vi "IMAQController.ImageProcessing.vi"(0 "i ref in":refnum<vi>, 1 "Image ref in":refnum<vi>, 2 "ActImage":T2, 3 "RawImage":T2, 4 "DIM data":i16[](array[numeric]), 5 "ImageHeight":i32, 6 "ImageWidth":i32, 7 "error in (no error)":errorcluster, 8 "Ana Step 1 Event":refnum<user-event>, 9 "Save?":bool, 10 "Grid Color":u32(colorbox)=16448250, 11 "Overlay Lines In":T4(array[cluster]), 12 "Save path in":path, 13 "Overlay already configured?":bool, 14 "Save Overlay?":bool, 15 "ShowGrid?":bool, 16 "Scan Variables":T1, 17 "SaveImage":T2, 18 "Scan Running?":bool, 19 "Averaging":u8=1) -> (20 "i ref out":refnum<vi>, 22 "Overlay Lines Out":T4(array[cluster]), 23 "ActImage Out":T2, 24 "Error?":bool, 25 "AverageString":string, 27 "error out":errorcluster)   [LabVIEW 2014, in "IMAQController.lvlib"]
uses:
  IMAQController.lvlib
  <vilib>/vision/Image Controls.llb/IMAQ Image.ctl
panel:
  out "activeCamera.Aqcuisation Mode":T3(ring)
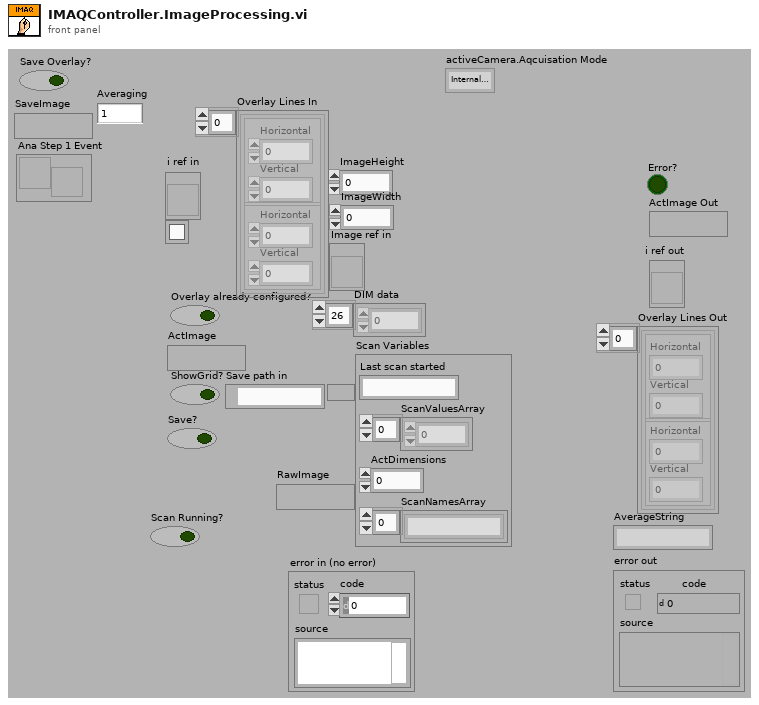
[diagram p1: front panel]
types:
  T1 = cluster{"Last scan started":string, "ScanValuesArray":dbl[], "ActDimensions":i16, "ScanNamesArray":string[]}
  T2 = typedef "IMAQ Image.ctl" = refnum<image>
  T3 = enum32{"Internal Trigger", "Scan", "free Running", "External Trigger"}
  T4 = cluster{cluster{"Horizontal":i32, "Vertical":i32}, cluster{"Horizontal":i32, "Vertical":i32}}[]
  T5 = enum32{"Gray", "Binary", "Gradient", "Rainbow", "Temperature"}
  T6 = typedef "IMAQController.lvlib/IMAQController.i attribute.ctl" = cluster{"ImageTakenID":i32, "actSequencer":string, "actScanner":string, "CameraTriggerID":i32, "activatedCameras":cluster{"Name":string, "Camera Type":string, "Acquisition Mode":u32, "JPEG Mode?":bool, "Acquisition Delay":dbl, "Save Images?":bool, "Center Coordinates":T7, "PixelPermm":cluster{"Horizontal":dbl, "Vertical":dbl}, "Rotation":dbl, "Mirror Mode":u32, "PixelCoordinates":cluster{"1":cluster{"Horizontal":i32, "Vertical":i32}, "2":cluster{"Horizontal":i32, "Vertical":i32}, "3":cluster{"Horizontal":i32, "Vertical":i32}, "4":cluster{"Horizontal":i32, "Vertical":i32}}, "RWCoordinates":cluster{"1":cluster{"Horizontal":dbl, "Vertical":dbl}, "2":cluster{"Horizontal":dbl, "Vertical":dbl}, "3":cluster{"Horizontal":dbl, "Vertical":dbl}, "4":cluster{"Horizontal":dbl, "Vertical":dbl}}, "HorizScaling":dbl, "VertScaling":dbl}[], "Ini C-Array":string[], "actCamera":string, "activeCamera":cluster{"Name":string, "Camera Type":string, "Aqcuisation Mode":enum32{"Internal Trigger", "Scan", "free Running", "External Trigger"}, "JPEG Mode?":bool, "Acquisition Delay":dbl, "Save Images?":bool, "Center Coordinates":T7, "PixelPermm":cluster{"Horizontal":dbl, "Vertical":dbl}, "Rotation":dbl, "Mirror Mode":u32, "PixelCoordinates":cluster{"1":cluster{"Horizontal":i32, "Vertical":i32}, "2":cluster{"Horizontal":i32, "Vertical":i32}, "3":cluster{"Horizontal":i32, "Vertical":i32}, "4":cluster{"Horizontal":i32, "Vertical":i32}}, "RWCoordinates":cluster{"1":cluster{"Horizontal":dbl, "Vertical":dbl}, "2":cluster{"Horizontal":dbl, "Vertical":dbl}, "3":cluster{"Horizontal":dbl, "Vertical":dbl}, "4":cluster{"Horizontal":dbl, "Vertical":dbl}}, "HorizScaling":dbl, "VertScaling":dbl}, "BilderMittelungen":u8, "OldPicture":dbl[][]}
  T7 = typedef "LVPoint32TypeDef.ctl" = cluster{"Horizontal":i32, "Vertical":i32}
  T8 = cluster{"Name":string, "Camera Type":string, "Acquisition Mode":u32, "JPEG Mode?":bool, "Acquisition Delay":dbl, "Save Images?":bool, "Center Coordinates":T7, "PixelPermm":cluster{"Horizontal":dbl, "Vertical":dbl}, "Rotation":dbl, "Mirror Mode":u32, "PixelCoordinates":cluster{"1":cluster{"Horizontal":i32, "Vertical":i32}, "2":cluster{"Horizontal":i32, "Vertical":i32}, "3":cluster{"Horizontal":i32, "Vertical":i32}, "4":cluster{"Horizontal":i32, "Vertical":i32}}, "RWCoordinates":cluster{"1":cluster{"Horizontal":dbl, "Vertical":dbl}, "2":cluster{"Horizontal":dbl, "Vertical":dbl}, "3":cluster{"Horizontal":dbl, "Vertical":dbl}, "4":cluster{"Horizontal":dbl, "Vertical":dbl}}, "HorizScaling":dbl, "VertScaling":dbl}[]
  T9 = cluster{"Name":string, "Camera Type":string, "Acquisition Mode":u32, "JPEG Mode?":bool, "Acquisition Delay":dbl, "Save Images?":bool, "Center Coordinates":T7, "PixelPermm":cluster{"Horizontal":dbl, "Vertical":dbl}, "Rotation":dbl, "Mirror Mode":u32, "PixelCoordinates":cluster{"1":cluster{"Horizontal":i32, "Vertical":i32}, "2":cluster{"Horizontal":i32, "Vertical":i32}, "3":cluster{"Horizontal":i32, "Vertical":i32}, "4":cluster{"Horizontal":i32, "Vertical":i32}}, "RWCoordinates":cluster{"1":cluster{"Horizontal":dbl, "Vertical":dbl}, "2":cluster{"Horizontal":dbl, "Vertical":dbl}, "3":cluster{"Horizontal":dbl, "Vertical":dbl}, "4":cluster{"Horizontal":dbl, "Vertical":dbl}}, "HorizScaling":dbl, "VertScaling":dbl}
  T10 = cluster{"Data":u8[][], "Height":i32, "Width":i32, "Save path out Scan":path, "Save path out Horizontal":path, "Save path out Vertical":path, "Scan?":bool, "Scan running?":bool, "ScanValuesArray":dbl[], "ActDimensions":i16, "ScanNamesArray":string[], "Av repeat?":bool}
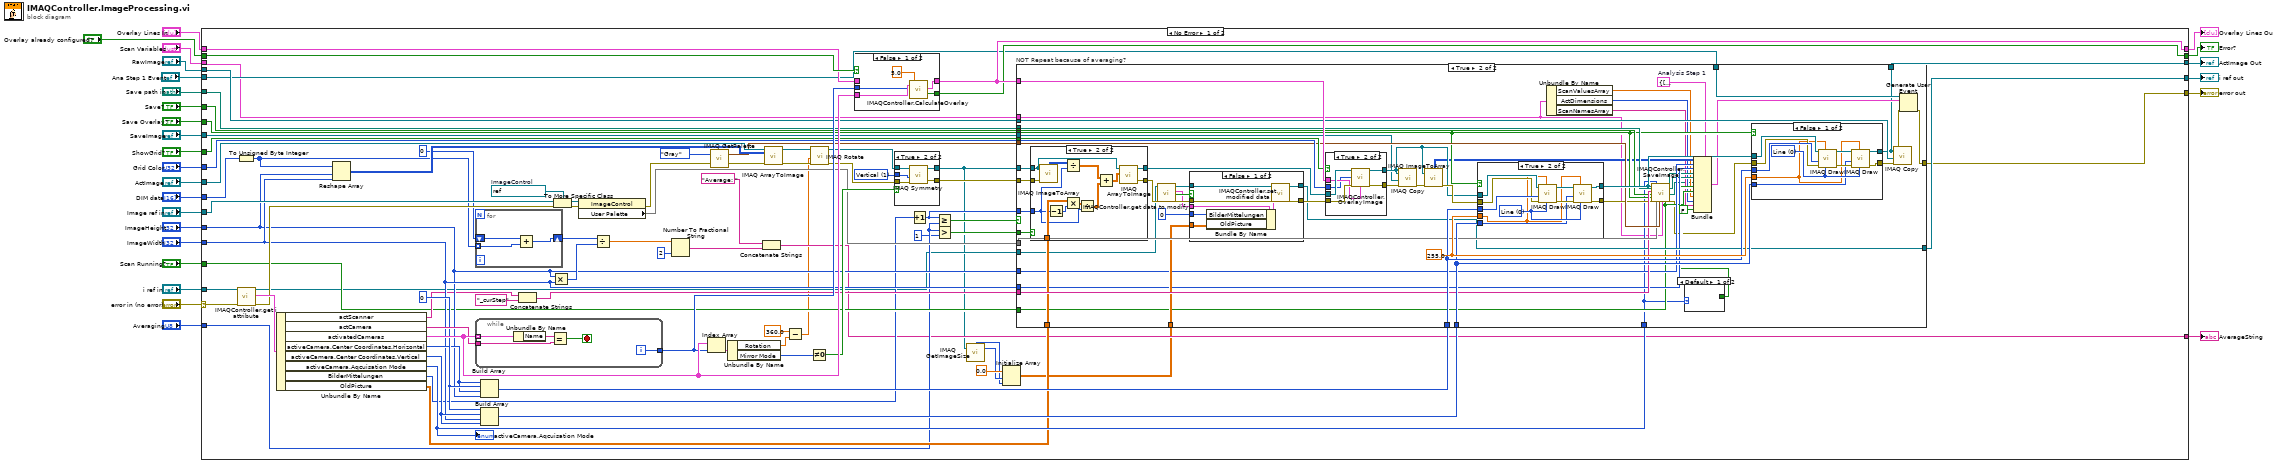
[diagram p0: block diagram]
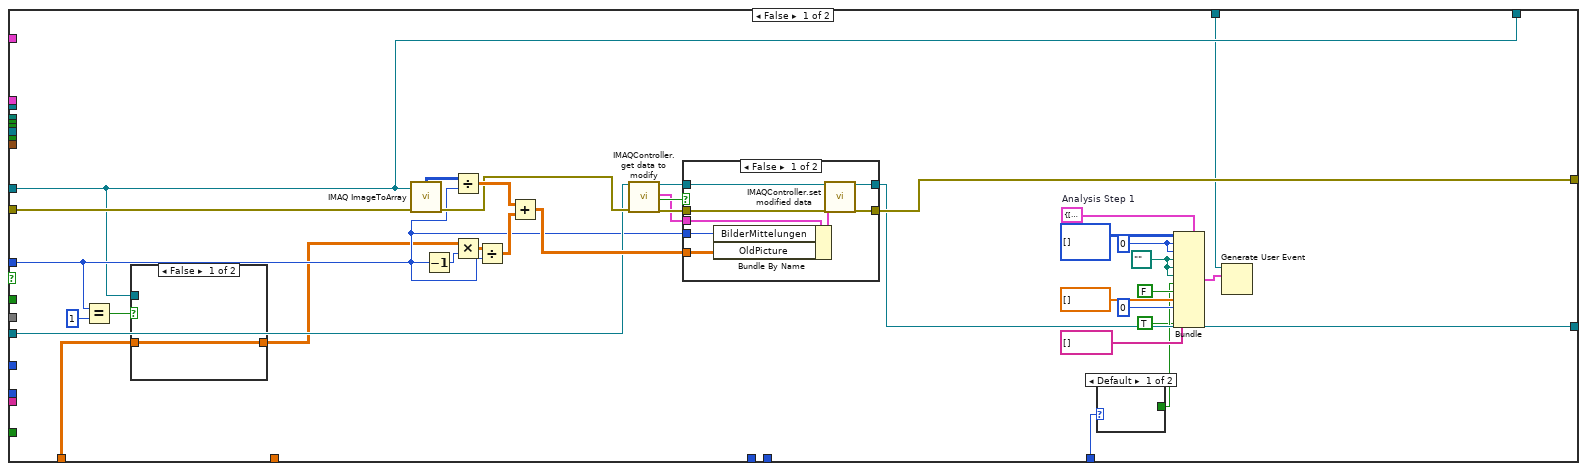
[diagram p2: hidden frame]
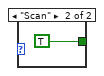
[diagram p3: hidden frame]
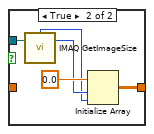
[diagram p4: hidden frame]
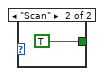
[diagram p6: hidden frame]
diagram:
  n1 = case shown="No Error" "error in (no error)" {
    selector: "error in (no error)" -> [w69 w297]
    tunnel: "i ref in" -> [w106 w296]
    tunnel: "Overlay already configured?" -> [w105 _]
    tunnel: "Overlay Lines In" -> [w104 _]
    tunnel: "Image ref in" -> [w103 _]
    tunnel: "DIM data" -> [w93 _]
    tunnel: "Grid Color" -> [w83 _]
    tunnel: [w82 _] -> w20
    tunnel: "ShowGrid?" -> [w81 _]
    tunnel: "Save path in" -> [w56 _]
    tunnel: "ImageHeight" -> [w61 _]
    tunnel: "ImageWidth" -> [w62 _]
    tunnel: [w39 _] -> w15
    tunnel: "RawImage" -> [w70 _]
    tunnel: [w32 w297] -> w13
    tunnel: "ActImage" -> [w68 w295]
    tunnel: [w33 w296] -> w10
    tunnel: [w59 w295] -> w9
    tunnel: "Save?" -> [w52 _]
    tunnel: [w66 _] -> w7
    tunnel: "Save Overlay?" -> [w51 _]
    tunnel: "SaveImage" -> [w49 _]
    tunnel: "Scan Variables" -> [w30 _]
    tunnel: "Scan Running?" -> [w48 _]
    tunnel: "Averaging" -> [w44 _]
    tunnel: "Ana Step 1 Event" -> [w31 _]
    frame No Error {
      w65 = 0 ("element")
      w87 = u32 1 items=["Horizontal", "Vertical", "Central", "1st Diagonal", "2nd Diagonal"] ("Type of Symmetry")
      w102 = refnum<vi> refnum  # ImageControl
      n2 = To Unsigned Byte Integer(number=w93) -> (unsigned 8bit integer=w71:u8[])
      n3 = call "IMAQController.get i attribute.vi"("i ref in"=w106, "error in (no error)"=w69) -> ("i ref out"=w40:refnum<vi>, "i attribute"=w107:T6, "error out"=w100:errorcluster)  [unwired: 15 in]
      n4 = Unbundle By Name(w107) -> ("actScanner"=w60:string, "actCamera"=w80:string, "activatedCameras"=w92:T8, "activeCamera.Center Coordinates.Horizontal"=w64:i32, "activeCamera.Center Coordinates.Vertical"=w63:i32, "activeCamera.Aqcuisation Mode"=w50:T3, "BilderMittelungen"=w45:u8, "OldPicture"=w46:dbl[][])
      "activeCamera.Aqcuisation Mode" <- w50
      n5 = Reshape Array(w71, w61, w62) -> (w94:u8[][])
      n6 = for {
        tunnel: w71 -> [w281] mode=indexing
        shift-right: [w280] -> w77
        shift-left: 0 -> [w282]
        n7 = Add(x=w282, y=w281) -> (x+y=w280:i32)
      }
      n8 = while {
        tunnel: w92 -> [w291] mode=indexing
        tunnel: w80 -> [w294]
        tunnel: [w292] -> w91
        i -> [w292]
        stop <- w293 stop-if-true
        n9 = Unbundle By Name(w291) -> ("Name"=w290:string)
        n10 = Equal?(x=w290, y=w294) -> (x = y?=w293:bool)
      }
      n11 = Build Array(w64, w65, w64, w61) -> (w58:i32[])
      n12 = Build Array(w65, w63, w62, w63) -> (w57:i32[])
      n13 = Concatenate Strings(w60, "_curStep" ("string")) -> (w53:string)
      n14 = Multiply(x=w61, y=w62) -> (x*y=w75:i32)
      n15 = To More Specific Class(target class=w102, reference=w103, error in=w100) -> (specific class reference=w101:refnum<vi>, error out=w99:errorcluster)
      n16 = property on="Property Node" class="ImageControl"(reference=w101, error in=w99) -> (error out=w97:errorcluster, "User Palette"=w54)  [unwired: 1 out]
      n17 = Divide(x=w77, y=w75) -> (x/y=w76:dbl)
      n18 = Number To Fractional String(number=w76, precision (6)=i16 2 ("width (-)")) -> (F-format string=w73:string)  [unwired: 2 in]
      n19 = Index Array(array=w92, index=w91) -> (element=w90:T9)
      n20 = call "IMAQ GetPalette"("Palette Number (gray)"=T5."Gray", "error in (no error)"=w97) -> ("Color Palette"=w55:cluster{"Red":u8, "Green":u8, "Blue":u8}[], "error out"=w96:errorcluster)  [unwired: 3 in]
      n21 = Unbundle By Name(w90) -> ("Rotation"=w28:dbl, "Mirror Mode"=w86:u32)
      n22 = Concatenate Strings("Average: " ("string"), w73) -> (w39:string)
      n23 = call "IMAQ ArrayToImage"("error in (no error)"=w96, "Image Pixels (U8)"=w94, "Image"=w68) -> ("error out"=w95:errorcluster, "Image Out"=w67:T2)  [unwired: 7 in]
      n24 = Subtract(x=360.0, y=w28) -> (x-y=w27:dbl)
      n25 = Not Equal To 0?(x=w86) -> (x != 0?=w85:bool)
      n26 = call "IMAQ Rotate"("error in (no error)"=w95, "Angle (degrees)"=w27, "Image Src"=w67) -> ("error out"=w88:errorcluster, "Image Dst Out"=w89:T2)  [unwired: 7 in]
      n27 = case shown="False" w105 {
        tunnel: w92 -> [w276 _]
        tunnel: [w277 w279] -> w82
        tunnel: w104 -> [_ w279]
        tunnel: w91 -> [w275 _]
        tunnel: [w274 _] -> w66
        frame False {
          n28 = call "IMAQController.CalculateOverlay.vi"("activatedCameras"=w276, "Select Camera"=w275, "Line Every mm"=5.0) -> ("Overlay Lines"=w277:T4, "Error?"=w274:bool)  [unwired: 15 in]
        }
        frame True {
        }
      }
      n29 = case shown="True" w85 {
        tunnel: w89 -> [w283 w287]
        tunnel: w88 -> [w284 w289]
        tunnel: [w284 w288] -> w84
        tunnel: [w283 w286] -> w35
        tunnel: w87 -> [_ w285]
        frame False {
        }
        frame True {
          n30 = call "IMAQ Symmetry"("error in (no error)"=w289, "Type of Symmetry"=w285, "Image Src"=w287) -> ("error out"=w288:errorcluster, "Image Dst Out"=w286:T2)  [unwired: 2 in]
        }
      }
      n31 = Increment(x=w45) -> (x+1=w41:u8)
      n32 = Greater Or Equal?(x=w41, y=w44) -> (x >= y?=w47:bool)
      n33 = Greater?(x=w44, y=u8 1) -> (0:w42:bool)
      n34 = call "IMAQ GetImageSize"("Image"=w35) -> ("Y Resolution"=w37:i32, "X Resolution"=w36:i32)  [unwired: 3 in, 1 out]
      n35 = Initialize Array(0.0, w37, w36) -> (w34:dbl[][])
      n36 = case "NOT Repeat because of averaging?" shown="True" w47 {
        tunnel: w35 -> [w124 w193]
        tunnel: w84 -> [w141 w192]
        tunnel: w83 -> [_ w216]
        tunnel: w82 -> [_ w215]
        tunnel: w81 -> [_ w214]
        tunnel: w70 -> [_ w213]
        tunnel: [w128 w159] -> w32
        tunnel: w62 -> [_ w176]
        tunnel: w61 -> [_ w175]
        tunnel: [w124 w165] -> w59
        tunnel: w58 -> [_ w209]
        tunnel: w57 -> [_ w208]
        tunnel: w56 -> [_ w206]
        tunnel: w55 -> [_ w205]
        tunnel: w54 -> [_ w204]
        tunnel: w53 -> [_ w203]
        tunnel: w52 -> [_ w202]
        tunnel: w51 -> [_ w201]
        tunnel: w50 -> [w111 w171]
        tunnel: w49 -> [_ w196]
        tunnel: w30 -> [_ w169]
        tunnel: w48 -> [_ w172]
        tunnel: w46 -> [w123 w191]
        tunnel: w42 -> [_ w195]
        tunnel: w41 -> [w127 w190]
        tunnel: w40 -> [w129 w186]
        tunnel: [w121 w184] -> w33
        tunnel: w34 -> [_ w180]
        tunnel: w31 -> [w119 w179]
        frame False {
          w109 = T10 {"Data"=[], "Height"=0, "Width"=0, "Save path out Scan"=path "", "Save path out Horizontal"=path "", "Save path out Vertical"=path "", "Scan?"=TRUE, "Scan running?"=TRUE, "ScanValuesArray"=[], "ActDimensions"=0, "ScanNamesArray"=[], "Av repeat?"=FALSE}  # Analysis Step 1
          w116 = path "" ("Save path out Scan")
          w117 = 0 ("Height")
          n37 = Equal?(x=w127, y=u8 1) -> (x = y?=w125:bool)
          n38 = case shown="False" w125 {
            tunnel: w124 -> [_ w148]
            tunnel: w123 -> [w143 _]
            tunnel: [w143 w147] -> w122
            frame False {
            }
            frame True {
              n39 = call "IMAQ GetImageSize"("Image"=w148) -> ("Y Resolution"=w145:i32, "X Resolution"=w144:i32)  [unwired: 3 in, 1 out]
              n40 = Initialize Array(0.0, w145, w144) -> (w147:dbl[][])
            }
          }
          n41 = call "IMAQ ImageToArray"("error in (no error)"=w141, "Image"=w124) -> ("error out"=w130:errorcluster, "Image Pixels (U8)"=w134:u8[][])  [unwired: 2 in, 3 out]
          n42 = Decrement(x=w127) -> (x-1=w136:u8)
          n43 = Divide(x=w134, y=w127) -> (x/y=w132:dbl[][])
          n44 = Multiply(x=w122, y=w136) -> (x*y=w135:dbl[][])
          n45 = Divide(x=w135, y=w127) -> (x/y=w133:dbl[][])
          n46 = Add(x=w132, y=w133) -> (x+y=w131:dbl[][])
          n47 = call "IMAQController.get data to modify.vi"("i ref in"=w129, "error in (no error)"=w130) -> ("i ref out"=w139:refnum<vi>, "i attribute"=w137:T6, "timed out"=w138:bool, "error out"=w140:errorcluster)  [unwired: 14 in]
          n48 = case shown="False" w138 {
            tunnel: [w156 w157] -> w128
            tunnel: w140 -> [w155 w157]
            tunnel: w139 -> [w154 w158]
            tunnel: [w153 w158] -> w121
            tunnel: w137 -> [w152 _]
            tunnel: w127 -> [w150 _]
            tunnel: w131 -> [w149 _]
            frame False {
              n49 = Bundle By Name(cluster=w152, "BilderMittelungen"=w150, "OldPicture"=w149) -> (w151:T6)
              n50 = call "IMAQController.set modified data.vi"("i ref in"=w154, "i attribute"=w151, "error in (no error)"=w155) -> ("i ref out"=w153:refnum<vi>, "error out"=w156:errorcluster)  [unwired: 15 in]
            }
            frame True {
            }
          }
          n51 = case shown="Default" w111 {
            tunnel: [_ TRUE] -> w110
            frame Default {
            }
            frame "Scan" {
            }
          }
          n52 = Bundle(cluster=w109, "Data"=u8[][] [], "Height"=w117, "Width"=w117, "Save path out Scan"=w116, "Save path out Horizontal"=w116, "Save path out Vertical"=w116, "Scan?"=w110, "Scan running?"=FALSE ("Scan?"), "ScanValuesArray"=dbl[] [], "ActDimensions"=i16 0, "ScanNamesArray"=string[] [], "Av repeat?"=TRUE) -> (w120:T10)
          n53 = Generate User Event(user event=w119, event data cluster=w120) -> ()  [unwired: 2 in, 2 out]
        }
        frame True {
          w163 = T10 {"Data"=[], "Height"=0, "Width"=0, "Save path out Scan"=path "", "Save path out Horizontal"=path "", "Save path out Vertical"=path "", "Scan?"=TRUE, "Scan running?"=TRUE, "ScanValuesArray"=[], "ActDimensions"=0, "ScanNamesArray"=[], "Av repeat?"=FALSE}  # Analysis Step 1
          w210 = sgl 255.0 ("Pixel Color")
          n54 = case shown="True" w195 {
            tunnel: [w229 w233] -> w194
            tunnel: w193 -> [w229 w230]
            tunnel: [w228 w232] -> w188
            tunnel: w192 -> [w228 w241]
            tunnel: w191 -> [_ w238]
            tunnel: w190 -> [_ w236]
            frame False {
            }
            frame True {
              n55 = call "IMAQ ImageToArray"("error in (no error)"=w241, "Image"=w230) -> ("Image Pixels (U8)"=w237:u8[][])  [unwired: 2 in, 4 out]
              n56 = Decrement(x=w236) -> (x-1=w240:u8)
              n57 = Divide(x=w237, y=w236) -> (x/y=w234:dbl[][])
              n58 = Multiply(x=w238, y=w240) -> (x*y=w239:dbl[][])
              n59 = Divide(x=w239, y=w236) -> (x/y=w235:dbl[][])
              n60 = Add(x=w234, y=w235) -> (x+y=w231:dbl[][])
              n61 = call "IMAQ ArrayToImage"("Image Pixels (U8)"=w231, "Image"=w230) -> ("error out"=w232:errorcluster, "Image Out"=w233:T2)  [unwired: 8 in]
            }
          }
          n62 = call "IMAQController.get data to modify.vi"("i ref in"=w186, "error in (no error)"=w188) -> ("i ref out"=w185:refnum<vi>, "i attribute"=w182:T6, "timed out"=w183:bool, "error out"=w187:errorcluster)  [unwired: 14 in]
          n63 = case shown="False" w183 {
            tunnel: [w225 w226] -> w189
            tunnel: w187 -> [w224 w226]
            tunnel: w185 -> [w223 w227]
            tunnel: [w222 w227] -> w184
            tunnel: w182 -> [w221 _]
            tunnel: w180 -> [w219 _]
            tunnel: u8 0 ("BilderMittelungen") -> [w218 _]
            frame False {
              n64 = Bundle By Name(cluster=w221, "BilderMittelungen"=w218, "OldPicture"=w219) -> (w220:T6)
              n65 = call "IMAQController.set modified data.vi"("i ref in"=w223, "i attribute"=w220, "error in (no error)"=w224) -> ("i ref out"=w222:refnum<vi>, "error out"=w225:errorcluster)  [unwired: 15 in]
            }
            frame True {
            }
          }
          n66 = case shown="True" w214 {
            tunnel: w194 -> [w267 w270]
            tunnel: [w267 w271] -> w197
            tunnel: w189 -> [w266 w273]
            tunnel: [w266 w272] -> w199
            tunnel: w215 -> [_ w269]
            tunnel: w216 -> [_ w268]
            frame False {
            }
            frame True {
              n67 = call "IMAQController.OverlayImage.vi"("Image In"=w270, "Color"=w268, "error in"=w273, "Overlay Lines"=w269) -> ("Image Out"=w271:T2, "error out"=w272:errorcluster)  [unwired: 14 in]
            }
          }
          n68 = call "IMAQ Copy"("error in (no error)"=w199, "Image Dst"=w196, "Image Src"=w197) -> ("error out"=w198:errorcluster)  [unwired: 3 in, 1 out]
          n69 = call "IMAQ ImageToArray"("error in (no error)"=w198, "Image"=w197) -> ("error out"=w212:errorcluster, "Image Pixels (U8)"=w177:u8[][])  [unwired: 2 in, 3 out]
          n70 = case shown="True" w201 {
            tunnel: w209 -> [_ w265]
            tunnel: w208 -> [_ w262]
            tunnel: w212 -> [w254 w260]
            tunnel: [w254 w259] -> w200
            tunnel: w197 -> [w255 w258]
            tunnel: [w255 w257] -> w207
            tunnel: w210 -> [_ w256]
            frame False {
            }
            frame True {
              w263 = u16 0 items=["Line", "Rectangle", "Oval"] ("Shape to draw")
              n71 = call "IMAQ Draw"("Shape to draw"=w263, "Pixel Color"=w256, "error in (no error)"=w260, "Coordinates"=w265, "Image Src"=w258) -> ("error out"=w264:errorcluster, "Image Dst Out"=w261:T2)  [unwired: 5 in]
              n72 = call "IMAQ Draw"("Shape to draw"=w263, "Pixel Color"=w256, "error in (no error)"=w264, "Coordinates"=w262, "Image Src"=w261) -> ("error out"=w259:errorcluster, "Image Dst Out"=w257:T2)  [unwired: 5 in]
            }
          }
          n73 = Unbundle By Name(w169) -> ("ScanValuesArray"=w168:dbl[], "ActDimensions"=w167:i16, "ScanNamesArray"=w166:string[])
          n74 = call "IMAQController.SaveImage.vi"("Image"=w207, "Save path in"=w206, "Service name"=w203, "Save?"=w202, "Save Overlay?"=w201, "error in"=w200, "Aqcuisation Mode"=w171, "User Palette"=w204, "Color Palette"=w205, "Scan Variables"=w169, "Scan Running?"=w172) -> ("Save path out Scan folder"=w173:path, "Save path out Horizontal"=w174:path, "Save path out Verical"=w164:path, "error out"=w161:errorcluster)  [unwired: 5 in]
          n75 = case shown="Default" w171 {
            tunnel: [_ TRUE] -> w170
            frame Default {
            }
            frame "Scan" {
            }
          }
          n76 = Bundle(cluster=w163, "Data"=w177, "Height"=w175, "Width"=w176, "Save path out Scan"=w173, "Save path out Horizontal"=w174, "Save path out Vertical"=w164, "Scan?"=w170, "Scan running?"=w172, "ScanValuesArray"=w168, "ActDimensions"=w167, "ScanNamesArray"=w166, "Av repeat?"=FALSE) -> (w178:T10)
          n77 = case shown="False" w201 {
            tunnel: w209 -> [w251 _]
            tunnel: w208 -> [w248 _]
            tunnel: w161 -> [w246 w252]
            tunnel: [w245 w252] -> w211
            tunnel: w207 -> [w244 w253]
            tunnel: [w243 w253] -> w165
            tunnel: w210 -> [w242 _]
            frame False {
              w249 = u16 0 items=["Line", "Rectangle", "Oval"] ("Shape to draw")
              n78 = call "IMAQ Draw"("Shape to draw"=w249, "Pixel Color"=w242, "error in (no error)"=w246, "Coordinates"=w251, "Image Src"=w244) -> ("error out"=w250:errorcluster, "Image Dst Out"=w247:T2)  [unwired: 5 in]
              n79 = call "IMAQ Draw"("Shape to draw"=w249, "Pixel Color"=w242, "error in (no error)"=w250, "Coordinates"=w248, "Image Src"=w247) -> ("error out"=w245:errorcluster, "Image Dst Out"=w243:T2)  [unwired: 5 in]
            }
            frame True {
            }
          }
          n80 = call "IMAQ Copy"("error in (no error)"=w211, "Image Dst"=w213, "Image Src"=w165) -> ("error out"=w160:errorcluster)  [unwired: 3 in, 1 out]
          n81 = Generate User Event(user event=w179, event data cluster=w178, error in=w160) -> (error out=w159:errorcluster)  [unwired: 1 in, 1 out]
        }
      }
    }
    frame Error {
    }
  }
  "Overlay Lines Out" <- w20
  "AverageString" <- w15
  "error out" <- w13
  "i ref out" <- w10
  "ActImage Out" <- w9
  "Error?" <- w7
